vi "Draw_Build Box Array.vi"(8 "Error":errorcluster, 11 "ICON Cluster":T4={"Header"="", "Body"=[], "ImageData"={"image type"=0, "image depth"=0, "image"=[], "mask"=[], "colors"=[], "Rectangle"={"left"=0, "top"=0, "right"=0, "bottom"=0}}, "New Icon"=bytes[0], "Line Status"=[], "Format"={"Color"={"Body txt"=255, "Body Back"=12632256, "Frame"=0, "Header txt"=32768, "Header Back"=16744703, "type"=enum."2 Color"}, "Icon Sizing"={"Rule"=enum."Static", "Header"=TRUE, "Rows"=5, "Width"=32, "Position"=enum."MID-CTR"}}} {"Format"."Icon Sizing"."Rows" min=1 max=5 step=1; "Format"."Icon Sizing"."Width" min=7 max=32 step=1}) -> (0 "Error Out":errorcluster, 2 "Fram Array Out":T1[](array[typedef]), 3 "ICON Cluster Out":T4={"Header"="", "Body"=[], "ImageData"={"image type"=0, "image depth"=0, "image"=[], "mask"=[], "colors"=[], "Rectangle"={"left"=0, "top"=0, "right"=0, "bottom"=0}}, "New Icon"=bytes[0], "Line Status"=[], "Format"={"Color"={"Body txt"=255, "Body Back"=12632256, "Frame"=0, "Header txt"=32768, "Header Back"=16744703, "type"=enum."2 Color"}, "Icon Sizing"={"Rule"=enum."Static", "Header"=TRUE, "Rows"=5, "Width"=32, "Position"=enum."MID-CTR"}}} {"Format"."Icon Sizing"."Rows" min=1 max=5 step=1; "Format"."Icon Sizing"."Width" min=7 max=32 step=1})   [LabVIEW 2009]
uses:
  Controls/Cluster/Cluster_Icon Data.ctl
  Controls/String_Picture/STRING_Line Display.ctl
  Controls/Array/String Array_Body Text.ctl
  Controls/Cluster/Cluster_Image Data.ctl
  Controls/Cluster/CLuster_Selectoin Box.ctl
  Controls/String_Picture/Picture_Icon.ctl
  Controls/Cluster/Cluster_Icon Format.ctl
  Controls/Cluster/Cluster_Icon Color Set.ctl
  Controls/Enum/ENUM_Frame Template Select.ctl
  Controls/Cluster/Cluster_Sizing Data.ctl
  Controls/Enum/ENUM_Icon Sizing.ctl
  Controls/Enum/RBENUM_Icon Position.ctl
  Controls/Cluster/Cluster_BOX Data.ctl
  Controls/Cluster/Cluster_Region info.ctl
  Controls/Cluster/Cluster_Top Left position.ctl
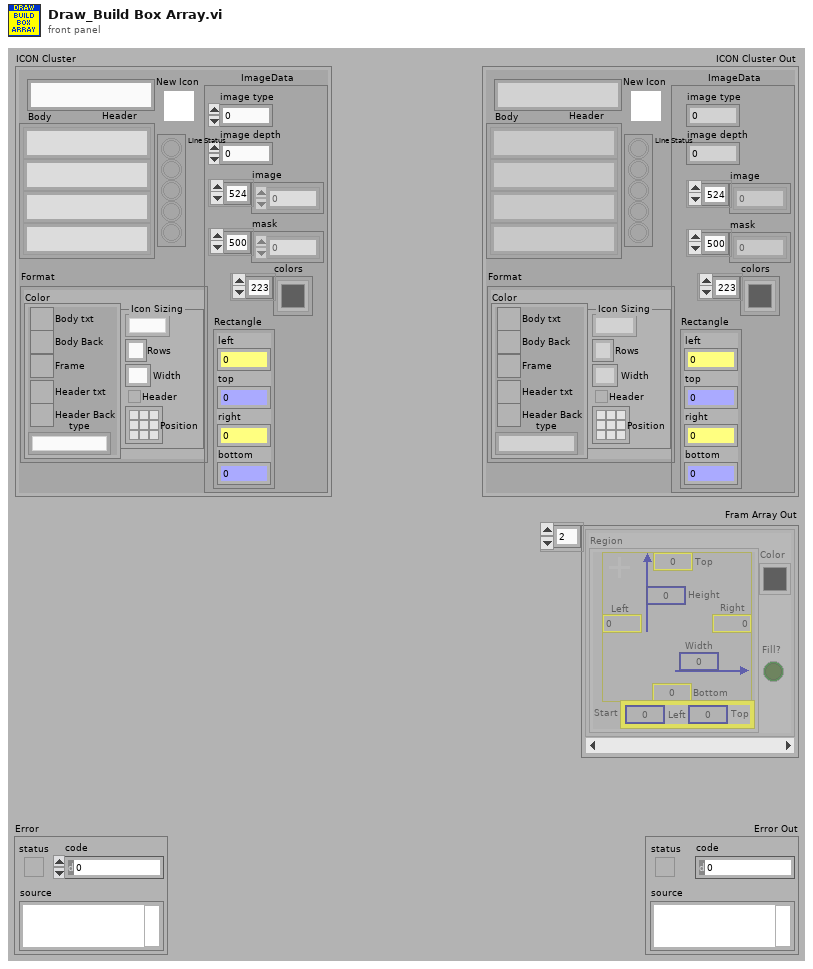
[diagram p1: front panel]
types:
  T1 = typedef "Cluster_BOX Data.ctl" = cluster{"Region":T2, "Color":u32, "Fill?":bool}
  T2 = typedef "Cluster_Region info.ctl" = cluster{"Left":i32, "Top":i32, "Right":i32, "Bottom":i32, "Width":u32, "Height":u32, "Start":T3}
  T3 = typedef "Cluster_Top Left position.ctl" = cluster{"Left":i32, "Top":i32}
  T4 = typedef "Cluster_Icon Data.ctl" = cluster{"Header":T5, "Body":T6, "ImageData":T7, "New Icon":T9, "Line Status":bool[], "Format":T10}
  T5 = typedef "STRING_Line Display.ctl" = string
  T6 = typedef "String Array_Body Text.ctl" = T5[]
  T7 = typedef "Cluster_Image Data.ctl" = cluster{"image type":i32, "image depth":i32, "image":u8[], "mask":u8[], "colors":u32[], "Rectangle":T8}
  T8 = typedef "CLuster_Selectoin Box.ctl" = cluster{"left":i16, "top":i16, "right":i16, "bottom":i16}
  T9 = typedef "Picture_Icon.ctl" = picture
  T10 = typedef "Cluster_Icon Format.ctl" = cluster{"Color":T11, "Icon Sizing":T13}
  T11 = typedef "Cluster_Icon Color Set.ctl" = cluster{"Body txt":u32, "Body Back":u32, "Frame":u32, "Header txt":u32, "Header Back":u32, "type":T12}
  T12 = typedef "ENUM_Frame Template Select.ctl" = enum16{"2 Color", "5 Color"}
  T13 = typedef "Cluster_Sizing Data.ctl" = cluster{"Rule":T14, "Header":bool, "Rows":u32, "Width":u32, "Position":T15}
  T14 = typedef "ENUM_Icon Sizing.ctl" = enum16{"Static", "Auto"}
  T15 = typedef "RBENUM_Icon Position.ctl" = enum32{"LFT-TOP", "MID-TOP", "RGT-TOP", "LFT-CTR", "MID-CTR", "RGT-CTR", "LFT-BOT", "MID-BOT", "RGT-BOT"}
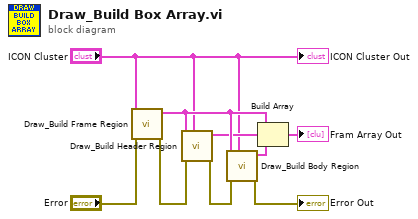
[diagram p0: block diagram]
diagram:
  n1 = call "Draw_Build Frame Region.vi"("Error"="Error", "ICON Cluster"="ICON Cluster") -> ("Error Out"=w4:errorcluster, "Frame Data Out"=w9:T1)  [unwired: 8 in]
  n2 = call "Draw_Build Header Region.vi"("ICON Cluster"="ICON Cluster", "Error"=w4, "Frame Data"=w9) -> ("Error Out"=w6:errorcluster, "Frame Data Out"=w8:T1)  [unwired: 7 in]
  n3 = call "Draw_Build Body Region.vi"("ICON Cluster"="ICON Cluster", "Error"=w6, "Frame Data"=w9) -> ("Error Out"=→"Error Out":errorcluster, "Frame Data Out"=w7:T1)  [unwired: 7 in]
  n4 = Build Array(w9, w8, w7) -> (→"Fram Array Out":T1[])
  "ICON Cluster Out" <- "ICON Cluster"
